vi "SDL Initialise.vi"(8 "error in (no error)":errorcluster) -> (0 "error out":errorcluster)   [LabVIEW 2021, in "Main Controller Actor.lvclass"]
uses:
  Main Controller Actor.lvclass
  LabSDL2/Source/Libraries/LibSDL2 Wrapper/Controls/Init Flags.ctl
  Globals.vi
  LabSDL2/Source/Libraries/LibSDL2 Wrapper/LibSDL2.lvlib
  LabSDL2/Source/Libraries/LibSDL2_Image Wrapper/LibSDL2_Image.lvlib
  LabSDL2/Source/Libraries/LibSDL2_TTF Wrapper/LibSDL2_TTF.lvlib
panel:
  out "appended path":path
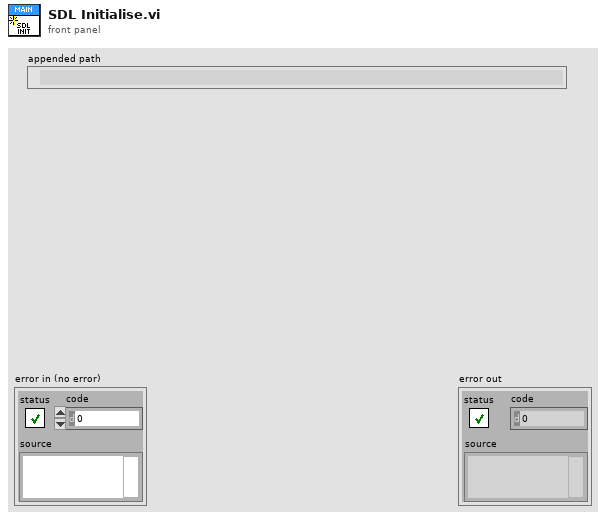
[diagram p1: front panel]
types:
  T1 = typedef "LibSDL2.lvlib/Init Flags.ctl" = u32
  T2 = typedef "Constants.ctl" = cluster{"Colours":cluster{"OK":u32, "Warning":u32, "Error":u32, "Red":u32, "Green":u32, "Blue":u32, "Yellow":u32}, "System":cluster{"Target Frames Second":dbl, "World Size":T3, "Window Size":T3, "Viewport Size":T3, "Sidebar Scaling":sgl, "Sidebar Width":i32, "SC2 Frame Rate [Seconds/Frame]":sgl}, "Game":cluster{"Maximum Asteroids":i32, "Max Energy":i32, "Max Crew":i32, "Maximum Stars":i32}}
  T3 = typedef "SDL2 Utility.lvlib/Point (I32).ctl" = cluster{"x":i32, "y":i32}
  T4 = cluster{"Renderer":u32, "Font":u32, "Window":u32, "Joystick":u32}
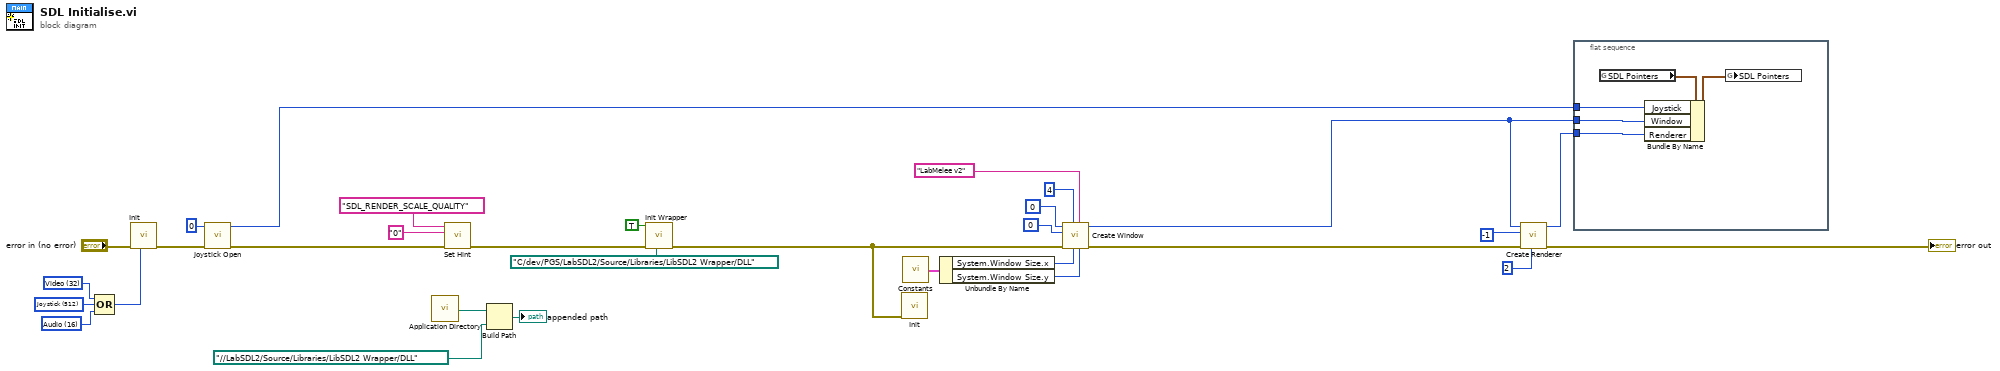
[diagram p0: block diagram]
diagram:
  w21 = T1 16 items=["Timer"=1, "Audio"=16, "Video"=32, "Joystick"=512, "Haptic"=4096, "Game Controller"=8192, "Events"=16384, "No Parachute"=1048576, "Everything"=17244689] ("Init Flags")
  w29 = T1 512 items=["Timer"=1, "Audio"=16, "Video"=32, "Joystick"=512, "Haptic"=4096, "Game Controller"=8192, "Events"=16384, "No Parachute"=1048576, "Everything"=17244689] ("Init Flags")
  w28 = T1 32 items=["Timer"=1, "Audio"=16, "Video"=32, "Joystick"=512, "Haptic"=4096, "Game Controller"=8192, "Events"=16384, "No Parachute"=1048576, "Everything"=17244689] ("Init Flags")
  n1 = Compound Arithmetic op=OR(w28, w29, w21) -> (w30:T1)
  n2 = call "Init.vi"("Flags"=w30, "error in"="error in (no error)") -> ("error out"=w31:errorcluster)  [unwired: 8 in, 1 out]
  n3 = call "Joystick Open.vi"("error in"=w31, "Device Index"=0) -> ("error out"=w10:errorcluster, "Joystick Pointer"=w11:u32)  [unwired: 8 in]
  n4 = call <vilib>:"Application Directory.vi"() -> ("Application Directory"=w3:path)
  n5 = call "Set Hint.vi"("error in"=w10, "Value"="0", "Name"="SDL_RENDER_SCALE_QUALITY") -> ("error out"=w23:errorcluster)  [unwired: 7 in, 1 out]
  n6 = Build Path(base path=w3, name or relative path=path "../../LabSDL2/Source/Libraries/LibSDL2 Wrapper/DLL" ("DLL Directory")) -> (appended path=→"appended path":path)
  n7 = call "Init Wrapper.vi"("DLL Directory"=path "C:/dev/PGS/LabSDL2/Source/Libraries/LibSDL2 Wrapper/DLL", "error in"=w23, "PNG (F)"=TRUE ("PNG")) -> ("error out"=w15:errorcluster)  [unwired: 7 in, 1 out]
  n8 = call "Init.vi"("error in (no error)"=w15) -> ()  [unwired: 9 in, 2 out]
  n9 = call "Constants.vi"() -> ("Constants"=w19:T2)
  n10 = Unbundle By Name(w19) -> ("System.Window Size.x"=w13:i32, "System.Window Size.y"=w12:i32)
  n11 = call "Create Window.vi"("Height"=w12, "Title"="LabMelee v2", "Width"=w13, "Flags"=u32 4, "error in"=w15, "Position y"=u32 0 ("Flags"), "Position x"=u32 0 ("Flags")) -> ("error out"=w8:errorcluster, "Window Pointer"=w6:u32)  [unwired: 3 in]
  n12 = call "Create Renderer.vi"("Flags"=u32 2, "error in"=w8, "Index"=-1, "Window Pointer"=w6) -> ("error out"=→"error out":errorcluster, "Renderer Pointer"=w9:u32)  [unwired: 6 in]
  n13 = flat-sequence {
    tunnel: w6 -> [w34]
    tunnel: w11 -> [w33]
    tunnel: w9 -> [w32]
    frame #0 {
      n14 = global read "Globals.vi" "SDL Pointers"() -> (w36:T4)
      n15 = Bundle By Name(cluster=w36, "Joystick"=w33, "Window"=w34, "Renderer"=w32) -> (w35:T4)
      n16 = global write "Globals.vi" "SDL Pointers"(w35) -> ()
    }
  }
